vi "LineToDirections.vi"(8 "MIN DISTANCE":bool, 9 "Line R":bool, 10 "Line C":bool, 11 "Line L":bool) -> (0 "STOP LINE":bool, 1 "Right":bool, 2 "Left":bool, 3 "Forward":bool)   [LabVIEW 2019]
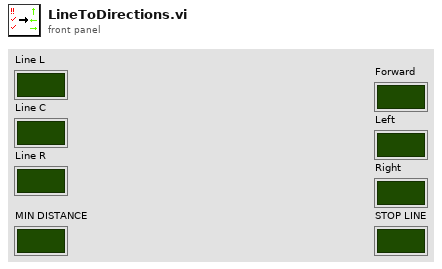
[diagram p1: front panel]
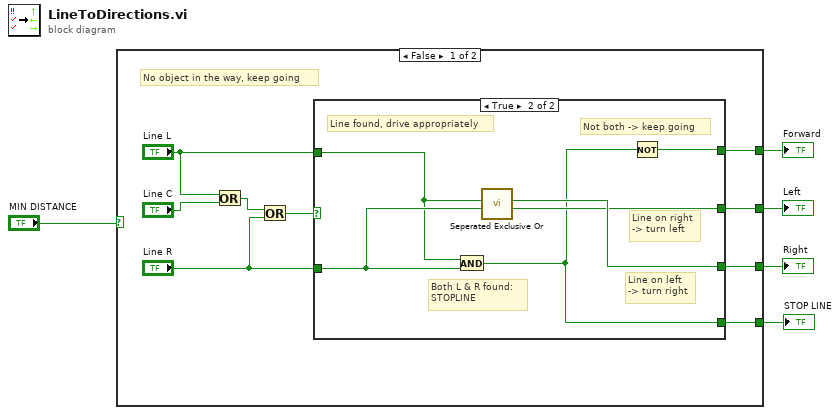
[diagram p0: block diagram]
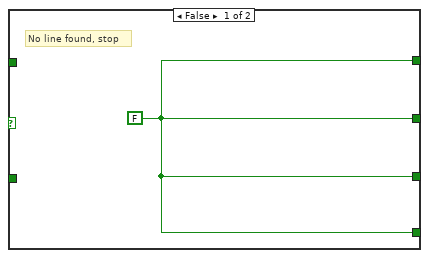
[diagram p2: hidden frame]
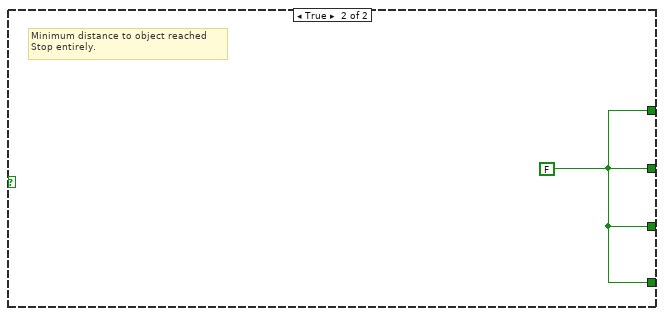
[diagram p3: hidden frame]
diagram:
  n1 = case shown="False" "MIN DISTANCE" {
    tunnel: [w14 w22] -> w5
    tunnel: [w13 w22] -> w4
    tunnel: [w12 w22] -> w3
    tunnel: [w6 w22] -> w1
    frame False {
      # "No object in the way, keep going"
      n2 = Or(x="Line L", y="Line C") -> (x .or. y?=w10:bool)
      n3 = Or(x=w10, y="Line R") -> (x .or. y?=w9:bool)
      n4 = case shown="True" w9 {
        tunnel: [w15 w20] -> w14
        tunnel: [w15 w17] -> w13
        tunnel: [w15 w21] -> w12
        tunnel: "Line R" -> [_ w19]
        tunnel: "Line L" -> [_ w18]
        tunnel: [w15 w16] -> w6
        frame False {
          w15 = FALSE
          # "No line found, stop"
        }
        frame True {
          # "Not both -> keep going"
          # "Both L & R found:\nSTOPLINE"
          # "Line on right\n-> turn left"
          # "Line on left\n-> turn right"
          # "Line found, drive appropriately"
          n5 = And(x=w18, y=w19) -> (x .and. y?=w16:bool)
          n6 = call "Seperated Exclusive Or.vi"("q"=w19, "p"=w18) -> ("only q"=w20:bool, "only p"=w21:bool)  [unwired: 8 in]
          n7 = Not(x=w16) -> (.not. x?=w17:bool)
        }
      }
    }
    frame True {
      w22 = FALSE
      # "Minimum distance to object reached\nStop entirely."
    }
  }
  "Forward" <- w4
  "Left" <- w5
  "Right" <- w3
  "STOP LINE" <- w1
